vi "Chroma_19020_Test.vi"(0 "VISA资源名称":refnum<visa-resource-name>, 5 "error in (no error)":errorcluster caption="错误输入（无错误）") -> (14 "VISA资源名称输出":refnum<visa-resource-name>, 15 "AC Tesult":string="116,116,116,116,116,116,116,116,112,112\r\n", 16 "IR Result":string="116,116,116,116,116,116,116,116,112,112\r\n", 18 "添加的数组":bool[][](array[boolean])=[[FALSE, FALSE, FALSE, FALSE, FALSE, FALSE, FALSE, FALSE], [TRUE, TRUE, TRUE, TRUE, TRUE, TRUE, TRUE, TRUE]], 19 "error out":errorcluster caption="错误输出")   [LabVIEW 2018]
uses:
  <vilib>/Instr/_visa.llb/VISA Configure Serial Port (Instr).vi
panel:
  out "IR Result数组":bool[](array[boolean])
  out "AC Tesult数组":bool[](array[boolean])
  out "数组 2":string[](array[string])
  out "数组":string[](array[string])
  out "读取缓冲区":string
  # "34,34,34,34,34,34,34,34,112,112"
  # "116,116,116,116,116,116,116,116,112,112"
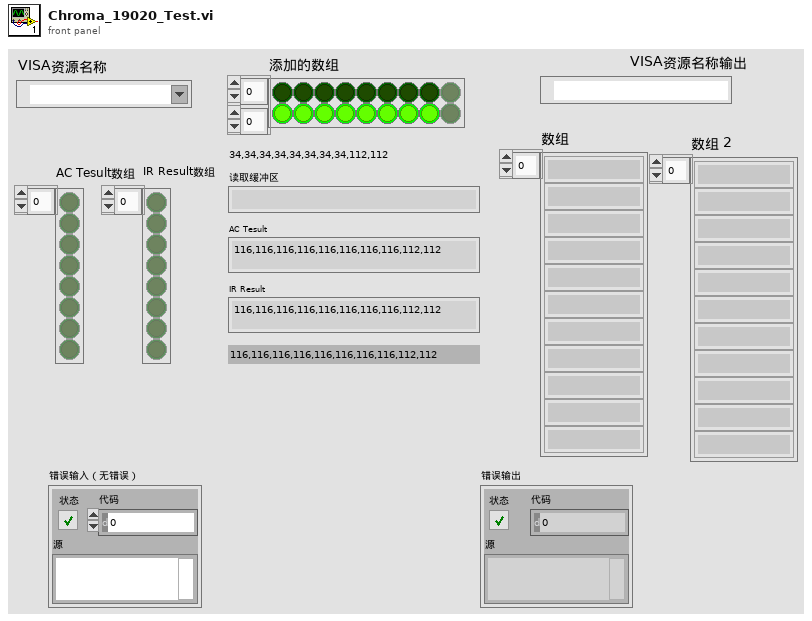
[diagram p1: front panel]
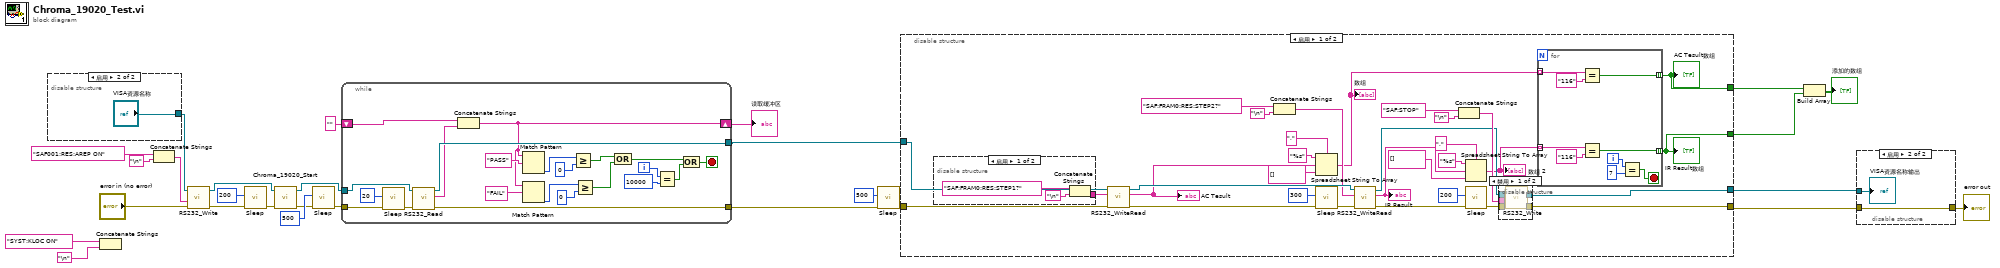
[diagram p0: block diagram]
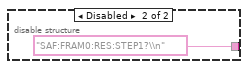
[diagram p2: hidden frame]
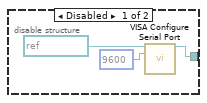
[diagram p5: hidden frame]
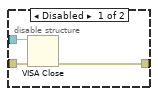
[diagram p6: hidden frame]
diagram:
  n1 = disable-structure shown="启用" {
    disable-tunnel: [w28 "VISA资源名称"] -> w24
    frame Disabled {
      n2 = call-poly "VISA Configure Serial Port"("VISA resource name"=refnum<visa-resource-name> "COM4", "baud rate (9600)"=u32 9600) -> ("VISA resource name out"=w28:refnum<visa-resource-name>)  [unwired: 12 in, 1 out]
    }
    frame Enabled {
    }
  }
  n3 = Concatenate Strings("SYST:KLOC ON" ("写入缓冲区"), "\n") -> ()  [unwired: 1 out]
  n4 = Concatenate Strings("SAF001:RES:AREP ON" ("写入缓冲区"), "\n") -> (w25:string)
  n5 = call "RS232_Write.vi"("错误输入（无错误）"="error in (no error)", "写入缓冲区"=w25, "VISA资源名称"=w24) -> ("错误输出"=w21:errorcluster, "VISA资源名称输出"=w23:refnum<visa-resource-name>)  [unwired: 7 in]
  n6 = call "Sleep.vi"("error in (no error)"=w21, "等待时间（毫秒）"=u32 200) -> ("error out"=w20:errorcluster)  [unwired: 9 in]
  n7 = call "Chroma_19020_Start.vi"("error in (no error)"=w20, "VISA引用句柄输入"=w23) -> ("error out"=w5:errorcluster, "VISA引用句柄输出"=w3:refnum<visa-resource-name>)  [unwired: 8 in]
  n8 = call "Sleep.vi"("error in (no error)"=w5, "等待时间（毫秒）"=u32 500) -> ("error out"=w4:errorcluster)  [unwired: 9 in]
  n9 = while {
    tunnel: w3 -> [w53]
    tunnel: [w52] -> w2
    tunnel: w4 -> [w49]
    tunnel: [w43] -> w1
    shift-right: [w38] -> w13
    shift-left: "" -> [w42]
    i -> [w48]
    stop <- w44 stop-if-true
    n10 = call "Sleep.vi"("error in (no error)"=w49, "等待时间（毫秒）"=u32 20) -> ("error out"=w50:errorcluster)  [unwired: 9 in]
    n11 = call "RS232_Read.vi"("错误输入（无错误）"=w50, "引用"=w53) -> ("错误输出"=w43:errorcluster, "读取缓冲区"=w41:string, "VISA资源名称输出"=w52:refnum<visa-resource-name>)  [unwired: 7 in]
    n12 = Concatenate Strings(w42, w41) -> (w38:string)
    n13 = Match Pattern(string=w38, regular expression="PASS" ("y")) -> (offset past match=w37:i32)  [unwired: 1 in, 3 out]
    n14 = Match Pattern(string=w38, regular expression="FAIL" ("y")) -> (offset past match=w34:i32)  [unwired: 1 in, 3 out]
    n15 = Greater Or Equal?(x=w37, y=0) -> (x >= y?=w32:bool)
    n16 = Greater Or Equal?(x=w34, y=0) -> (x >= y?=w33:bool)
    n17 = Compound Arithmetic op=OR ("复合运算")(w32, w33) -> (w45:bool)
    n18 = Equal?(x=w48, y=10000) -> (x = y?=w46:bool)
    n19 = Compound Arithmetic op=OR ("复合运算")(w45, w46) -> (w44:bool)
  }
  "读取缓冲区" <- w13
  n20 = call "Sleep.vi"("error in (no error)"=w1, "等待时间（毫秒）"=u32 500) -> ("error out"=w10:errorcluster)  [unwired: 9 in]
  n21 = disable-structure shown="启用" {
    disable-tunnel: w2 -> [w84 w106]
    disable-tunnel: [w80 w106] -> w12
    disable-tunnel: [w77 w105] -> w11
    disable-tunnel: w10 -> [w76 w105]
    disable-tunnel: [w56 _] -> w9
    disable-tunnel: [w55 _] -> w8
    frame Enabled {
      n22 = disable-structure shown="启用" {
        disable-tunnel: [w85 "SAF:FRAM0:RES:STEP1?\\n" ("写入缓冲区")] -> w54
        frame Enabled {
          n23 = Concatenate Strings("SAF:FRAM0:RES:STEP1?" ("写入缓冲区"), "\n") -> (w85:string)
        }
        frame Disabled {
        }
      }
      n24 = call "RS232_WriteRead.vi"("错误输入（无错误）"=w76, "写入缓冲区"=w54, "VISA资源名称"=w84) -> ("错误输出"=w78:errorcluster, "读取缓冲区"=w64:string, "VISA资源名称输出"=w71:refnum<visa-resource-name>)  [unwired: 6 in]
      "AC Tesult" <- w64
      n25 = Concatenate Strings("SAF:FRAM0:RES:STEP2?" ("写入缓冲区"), "\n") -> (w67:string)
      n26 = Spreadsheet String To Array(delimiter (Tab)="," ("分隔符(Tab)"), format string="%s" ("电子表格字符串"), spreadsheet string=w64, array type (2D Dbl)=string[] []) -> (array=w58:string[])
      "数组" <- w58
      n27 = call "Sleep.vi"("error in (no error)"=w78, "等待时间（毫秒）"=u32 300) -> ("error out"=w68:errorcluster)  [unwired: 9 in]
      n28 = call "RS232_WriteRead.vi"("错误输入（无错误）"=w68, "写入缓冲区"=w67, "VISA资源名称"=w71) -> ("错误输出"=w69:errorcluster, "读取缓冲区"=w60:string, "VISA资源名称输出"=w70:refnum<visa-resource-name>)  [unwired: 6 in]
      "IR Result" <- w60
      n29 = Concatenate Strings("SAF:STOP" ("写入缓冲区"), "\n") -> (w81:string)
      n30 = Spreadsheet String To Array(delimiter (Tab)="," ("分隔符(Tab)"), format string="%s" ("电子表格字符串"), spreadsheet string=w60, array type (2D Dbl)=string[] []) -> (array=w57:string[])
      "数组 2" <- w57
      n31 = call "Sleep.vi"("error in (no error)"=w69, "等待时间（毫秒）"=u32 200) -> ("error out"=w72:errorcluster)  [unwired: 9 in]
      n32 = disable-structure shown="禁用" {
        disable-tunnel: w81 -> [w93 _]
        disable-tunnel: [w92 w95] -> w80
        disable-tunnel: [w91 w94] -> w77
        disable-tunnel: w72 -> [w90 w94]
        disable-tunnel: w70 -> [w89 w95]
        frame Disabled {
          n33 = call "RS232_Write.vi"("错误输入（无错误）"=w90, "写入缓冲区"=w93, "VISA资源名称"=w89) -> ("错误输出"=w91:errorcluster, "VISA资源名称输出"=w92:refnum<visa-resource-name>)  [unwired: 7 in]
        }
        frame Enabled {
        }
      }
      n34 = for {
        tunnel: w58 -> [w101] mode=indexing
        tunnel: w57 -> [w98] mode=indexing
        tunnel: [w97] -> w55 mode=indexing
        tunnel: [w96] -> w56 mode=indexing
        i -> [w103]
        stop <- w102 stop-if-true
        n35 = Equal?(x=w101, y="116") -> (x = y?=w96:bool)
        n36 = Equal?(x=w98, y="116") -> (x = y?=w97:bool)
        n37 = Equal?(x=w103, y=7) -> (x = y?=w102:bool)
      }
      "AC Tesult数组" <- w56
      "IR Result数组" <- w55
    }
    frame Disabled {
    }
  }
  n38 = Build Array(w9, w8) -> (→"添加的数组":bool[][])
  n39 = disable-structure shown="启用" {
    disable-tunnel: w12 -> [w109 w111]
    disable-tunnel: w11 -> [w108 w110]
    disable-tunnel: [w107 w110] -> w16
    frame Disabled {
      n40 = VISA Close(VISA resource name=w109, error in (no error)=w108) -> (error out=w107:errorcluster)
    }
    frame Enabled {
      "VISA资源名称输出" <- w111
    }
  }
  "error out" <- w16
